vi "small_Desktop Main.vi"() -> ()   [LabVIEW 2019]
doc: "Demonstrates the use of the Network Streams functions to send LED status to the myRIO target."
uses:
  <vilib>/ErrorRing/Error Ring.xnode
panel:
  in  "Direction":dbl
  in  "Frequency":dbl
  in  "Enable":bool
  out "Array":dbl[](array[numeric])
  out "loops":i32
  in  "Stop":bool
  out "error out":errorcluster
  in  "Target IP Address":string="172.22.11.2"
  # "Overview: Magnetic field calculation, and send parameters to myRIO\nInstructions:\n1. Verify the value of Target IP Address. Set Visa resource name.\n2. Ensure RT Main.vi is already running. \n3. Run this VI. Set parameters of magnetic field."
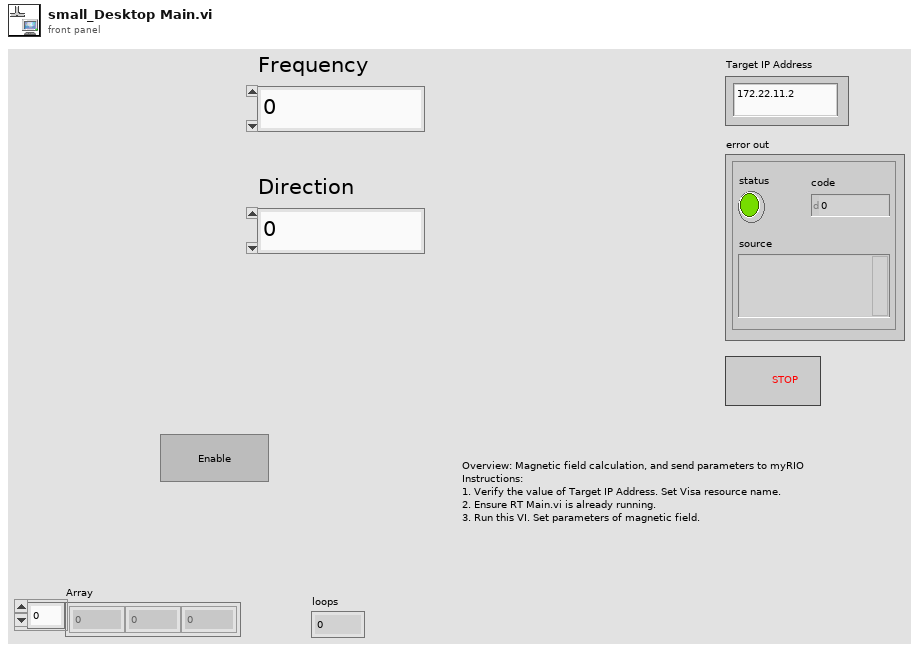
[diagram p1: front panel]
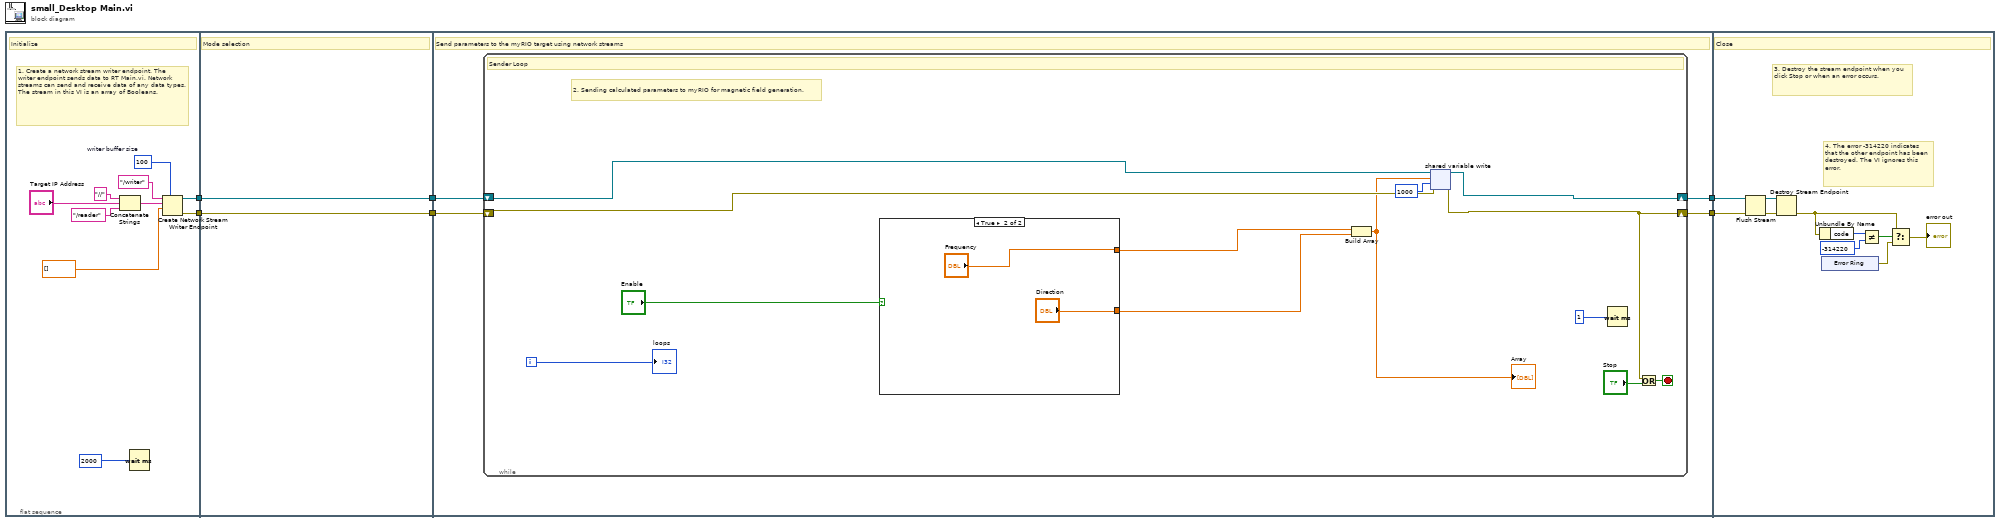
[diagram p0: block diagram]
diagram:
  n1 = flat-sequence {
    tunnel: [w11] -> w2
    tunnel: [w10] -> w1
    tunnel: [w18] -> w4
    tunnel: [w17] -> w3
    tunnel: w1 -> [w17]
    tunnel: w2 -> [w18]
    tunnel: [w20] -> w6
    tunnel: w4 -> [w22]
    tunnel: [w19] -> w5
    tunnel: w3 -> [w21]
    tunnel: w6 -> [w47]
    tunnel: w5 -> [w44]
    frame #0 {
      w9 = 100  # writer buffer size
      # "1. Create a network stream writer endpoint. The writer endpoint sends data to RT Main.vi. Network streams can send and receive data of any data types. The stream in this VI is an array of Booleans."
      # "Initialize"
      n2 = Concatenate Strings("//", "Target IP Address", "/reader") -> (w16:string)
      n3 = Wait (ms)(milliseconds to wait=2000) -> ()  [unwired: 1 out]
      n4 = Create Network Stream Writer Endpoint(7:w9, 9:dbl[] [], 10:w16, 11:"/writer" ("reader name")) -> (0:w10:errorcluster, 3:w11:refnum<k21>)  [unwired: 3 in]
    }
    frame #1 {
      # "Mode selection"
    }
    frame #2 {
      # "Send parameters to the myRIO target using network streams"
      n5 = while {
        shift-right: [w29] -> w19
        shift-left: w21 -> [w31]
        shift-right: [w30] -> w20
        shift-left: w22 -> [w32]
        i -> [w28]
        stop <- w35 stop-if-true
        # "2. Sending calculated parameters to myRIO for magnetic field generation."
        # "Sender Loop"
        n6 = case shown="True" "Enable" {
          tunnel: [_ "Frequency"] -> w26
          tunnel: [_ "Direction"] -> w25
          frame False {
          }
          frame True {
          }
        }
        n7 = Build Array ("创建数组")(w26, w25) -> (w24:dbl[])
        "Array" <- w24
        n8 = shared-variable-write(w32, w31, w24, 1000 ("timeout ms (-1)")) -> (w30:refnum<k21>, w29:errorcluster)  [unwired: 1 out]
        n9 = Wait (ms)(milliseconds to wait=u32 1) -> ()  [unwired: 1 out]
        n10 = Or(x=w29, y="Stop") -> (x .or. y?=w35:bool)
        "loops" <- w28
      }
    }
    frame #3 {
      # "4. The error -314220 indicates that the other endpoint has been destroyed. The VI ignores this error."
      # "3. Destroy the stream endpoint when you click Stop or when an error occurs."
      # "Close"
      n11 = Flush Stream(8:w44, 11:w47) -> (0:w45:errorcluster, 3:w46:refnum<k21>)  [unwired: 2 in, 1 out]
      n12 = Destroy Stream Endpoint(8:w45, 11:w46) -> (0:w39:errorcluster)
      n13 = Unbundle By Name(w39) -> ("code"=w43:i32)
      n14 = xnode "Error Ring"() -> ("error out"=w40:errorcluster)
      n15 = Not Equal?(x=w43, y=-314220) -> (x != y?=w41:bool)
      n16 = Select(t=w39, s=w41, f=w40) -> (s? t:f=→"error out":errorcluster)
    }
  }
